vi "Load DAC Configuration.vi"(8 "error in":errorcluster, 10 "Config File refnum in":T1, 11 "DAC HeatFlow AOV in":refnum<class "DAC HeatFlow AOV.lvclass">) -> (0 "error out":errorcluster, 2 "Config File refnum out":T1, 3 "DAC HeatFlow AOV out":refnum<class "DAC HeatFlow AOV.lvclass">)   [LabVIEW 2019, in "DAC.lvlib" / "DAC HeatFlow AOV.lvclass"]
uses:
  DAC HeatFlow AOV.lvclass
  C:/Users/krio/Documents/LV_Projects/test-stand/App/DAC/DAC.lvclass
  <vilib>/Utility/config.llb/Config Data RefNum.ctl
  DAC.lvclass/DAC.ctl
  DAC HeatFlow AOV.lvclass/DAC HeatFlow AOV.ctl
  <vilib>/Utility/config.llb/Read Key (String).vi
  DAC.lvclass
  <vilib>/Utility/config.llb/NI_LVConfig.lvlib
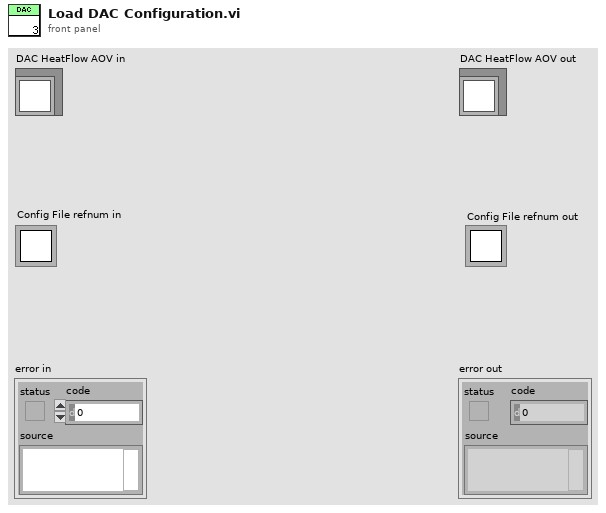
[diagram p1: front panel]
types:
  T1 = typedef "NI_LVConfig.lvlib/Config Data RefNum.ctl" = refnum<k1>
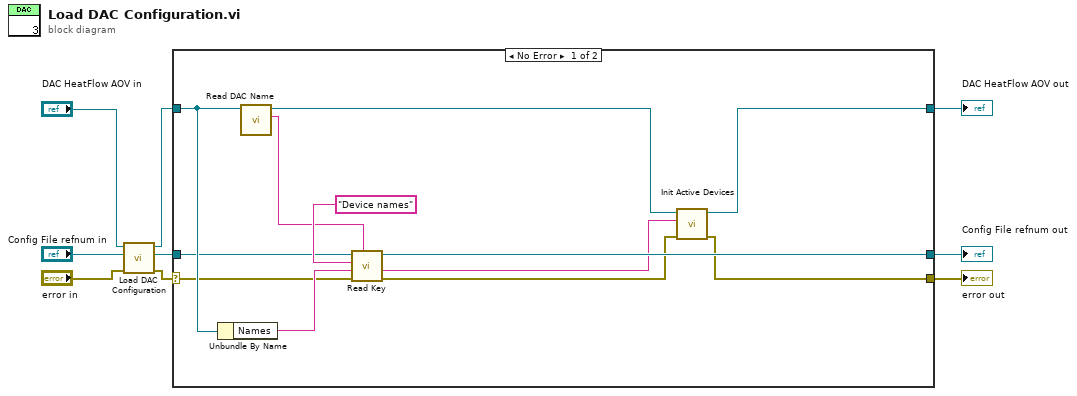
[diagram p0: block diagram]
diagram:
  n1 = call-parent "Load DAC Configuration.vi"("error in"="error in", "Config File refnum in"="Config File refnum in", "DAC in"="DAC HeatFlow AOV in") -> ("error out"=w4:errorcluster, "Config File refnum out"=w5:T1, "DAC out"=w6:refnum<class "DAC HeatFlow AOV.lvclass">)  [unwired: 6 in]
  n2 = case shown="No Error" w4 {
    selector: w4 -> [w10 w24]
    tunnel: [w13 w24] -> w1
    tunnel: [w16 w23] -> w3
    tunnel: w6 -> [w19 w23]
    tunnel: w5 -> [w11 w22]
    tunnel: [w21 w22] -> w2
    frame No Error {
      n3 = Unbundle By Name(w19) -> ("Names"=w18:string)
      n4 = call "Read DAC Name.vi"("DAC in"=w19) -> ("DAC Name"=w12:string, "DAC out"=w17:refnum<class "DAC HeatFlow AOV.lvclass">)  [unwired: 8 in, 1 out]
      n5 = call-poly <vilib>:"Read Key.vi"("section"=w12, "error in (no error)"=w10, "default value"=w18, "key"="Device names", "refnum"=w11) -> ("error out"=w14:errorcluster, "value"=w15:string, "refnum out"=w21:T1)  [unwired: 3 in, 1 out]
      n6 = call "Init Active Devices.vi"("error in"=w14, "Device Names"=w15, "DAC HeatFlow AIV in"=w17) -> ("error out"=w13:errorcluster, "DAC HeatFlow AIV out"=w16:refnum<class "DAC HeatFlow AOV.lvclass">)  [unwired: 7 in]
    }
    frame Error {
    }
  }
  "error out" <- w1
  "DAC HeatFlow AOV out" <- w3
  "Config File refnum out" <- w2
